vi "Keithley2200series_Write.vi"(0 "VISA resource name 2":refnum<visa-resource-name>, 1 "Function(0:Voltage) 3":u16(ring) items=["Voltage", "Current"], 2 "Out set 2":dbl, 3 "error in (no error)":errorcluster, 4 "Cml set 2":dbl) -> (5 "VISA out":refnum<visa-resource-name>, 6 "Meas Func":i32, 7 "error out 2":errorcluster)   [LabVIEW 2014]
uses:
  C:/Users/rad/Desktop/Keithley 2200 Series Power Supplies Ver 1.2 (LV2009)/Keithley 2200 Series/Keithley 2200 Series.lvlib
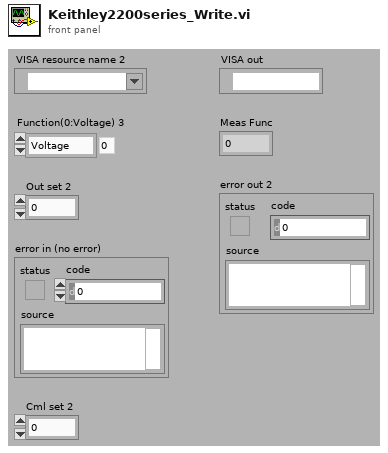
[diagram p1: front panel]
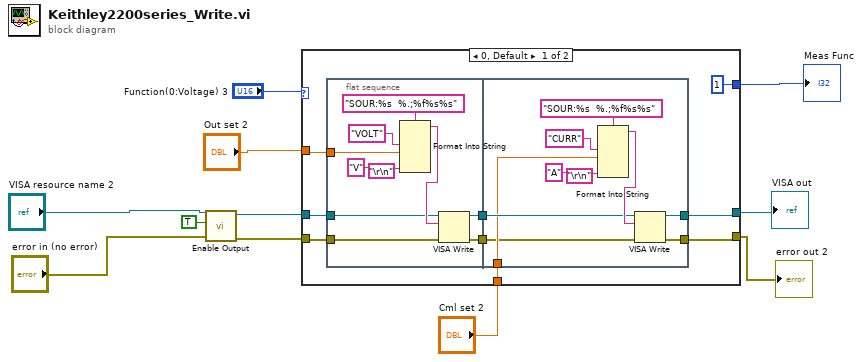
[diagram p0: block diagram]
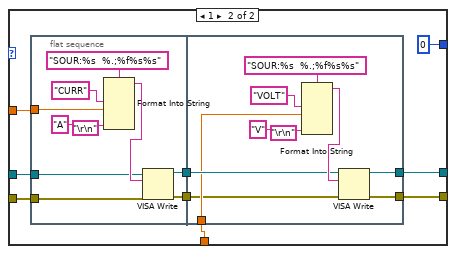
[diagram p2: hidden frame]
diagram:
  n1 = call "Enable Output.vi"("error in (no error)"="error in (no error)", "Enable Output (T: Enable)"=TRUE, "VISA resource name"="VISA resource name 2") -> ("error out"=w5:errorcluster, "VISA resource name out"=w6:refnum<visa-resource-name>)  [unwired: 7 out]
  n2 = case shown="0, Default" "Function(0:Voltage) 3" {
    tunnel: "Out set 2" -> [w20 w47]
    tunnel: "Cml set 2" -> [w18 w46]
    tunnel: w6 -> [w13 w45]
    tunnel: w5 -> [w12 w44]
    tunnel: [w16 w43] -> w4
    tunnel: [w15 w42] -> w3
    tunnel: [1 0] -> w11
    frame 0, Default {
      n3 = flat-sequence {
        tunnel: w20 -> [w28]
        tunnel: [w24] -> w19
        tunnel: [w23] -> w17
        tunnel: w13 -> [w22]
        tunnel: w12 -> [w21]
        tunnel: w19 -> [w35]
        tunnel: w18 -> [w34]
        tunnel: w17 -> [w33]
        tunnel: [w32] -> w16
        tunnel: [w31] -> w15
        frame #0 {
          n4 = Format Into String(format string="SOUR:%s  %.;%f%s%s", "VOLT" ("format string"), w28, "V" ("input 3"), "\r\n" ("End of Line Constant")) -> (resulting string=w25:string)  [unwired: 2 in, 1 out]
          n5 = VISA Write(VISA resource name=w22, write buffer=w25, error in (no error)=w21) -> (VISA resource name out=w24:refnum<visa-resource-name>, error out=w23:errorcluster)  [unwired: 1 out]
        }
        frame #1 {
          n6 = Format Into String(format string="SOUR:%s  %.;%f%s%s", "CURR" ("format string"), w34, "A" ("input 3"), "\r\n" ("End of Line Constant")) -> (resulting string=w36:string)  [unwired: 2 in, 1 out]
          n7 = VISA Write(VISA resource name=w35, write buffer=w36, error in (no error)=w33) -> (VISA resource name out=w32:refnum<visa-resource-name>, error out=w31:errorcluster)  [unwired: 1 out]
        }
      }
    }
    frame 1 {
      n8 = flat-sequence {
        tunnel: w47 -> [w57]
        tunnel: [w53] -> w49
        tunnel: [w52] -> w48
        tunnel: w45 -> [w51]
        tunnel: w44 -> [w50]
        tunnel: w49 -> [w64]
        tunnel: w46 -> [w63]
        tunnel: w48 -> [w62]
        tunnel: [w61] -> w43
        tunnel: [w60] -> w42
        frame #0 {
          n9 = Format Into String(format string="SOUR:%s  %.;%f%s%s", "CURR" ("format string"), w57, "A" ("input 3"), "\r\n" ("End of Line Constant")) -> (resulting string=w54:string)  [unwired: 2 in, 1 out]
          n10 = VISA Write(VISA resource name=w51, write buffer=w54, error in (no error)=w50) -> (VISA resource name out=w53:refnum<visa-resource-name>, error out=w52:errorcluster)  [unwired: 1 out]
        }
        frame #1 {
          n11 = Format Into String(format string="SOUR:%s  %.;%f%s%s", "VOLT" ("format string"), w63, "V" ("input 3"), "\r\n" ("End of Line Constant")) -> (resulting string=w65:string)  [unwired: 2 in, 1 out]
          n12 = VISA Write(VISA resource name=w64, write buffer=w65, error in (no error)=w62) -> (VISA resource name out=w61:refnum<visa-resource-name>, error out=w60:errorcluster)  [unwired: 1 out]
        }
      }
    }
  }
  "VISA out" <- w4
  "error out 2" <- w3
  "Meas Func" <- w11
